vi "Finish.vi"   [LabVIEW 2015]
doc: "This VI is called just before exiting. It is expected to close I/O refnum, save collected data, etc."
uses:
  <vilib>/Rock Robotics/WPI/Utilities/WPI_GetSetVariantRefNum.vi
types:
  T1 = typedef "WPI_JoystickDevRef.ctl" = cluster{"Device":T2}
  T2 = typedef "WPI_JoystickDeviceEnum.ctl" = enum16{"USB 0", "USB 1", "USB 2", "USB 3", "USB 4", "USB 5"}
  T3 = typedef "WPI_CompressorDevRef.ctl" = cluster{"DevStatus":errorcluster, "Pneumatics Control Module":u8}
  T4 = typedef "WPI_EncoderDevRef.ctl" = cluster{"DevStatus":errorcluster, "EncoderIndex":T5, "CounterIndex":T6, "DistancePerCount":dbl, "Decoding Type":T7}
  T5 = typedef "FPGA_EncoderIdx.ctl" = enum8{"Enc 0", "Enc 1", "Enc 2", "Enc 3", "Enc 4", "Enc 5", "Enc 6", "Enc 7", "Invalid"}
  T6 = typedef "FPGA_CounterCtrSystemIndex.ctl" = enum8{"Ctr 0", "Ctr 1", "Ctr 2", "Ctr 3", "Ctr 4", "Ctr 5", "Ctr 6", "Ctr 7", "Invalid"}
  T7 = typedef "WPI_EncoderType.ctl" = enum16{"1x", "2x", "4x"}
  T8 = typedef "WPI_SolenoidDevRef.ctl" = cluster{"DevStatus":errorcluster, "Pneumatics Control Module":u8, "Forward Solenoid Channel":T9, "Reverse Solenoid Channel":T9}
  T9 = typedef "WPI_SolenoidChannel.ctl" = enum8{"Solenoid 0", "Solenoid 1", "Solenoid 2", "Solenoid 3", "Solenoid 4", "Solenoid 5", "Solenoid 6", "Solenoid 7", "Invalid"}
  T10 = typedef "WPI_ServoDeviceRef.ctl" = cluster{"DeviceStatus":errorcluster, "PWM Channel":T11, "DeadBand":T12}
  T11 = typedef "FPGA_DIOPWMChannel.ctl" = enum8{"PWM 0", "PWM 1", "PWM 2", "PWM 3", "PWM 4", "PWM 5", "PWM 6", "PWM 7", "PWM 8", "PWM 9", "PWM MXP 0", "PWM MXP 1", "PWM MXP 2", "PWM MXP 3", "PWM MXP 4", "PWM MXP 5", "PWM MXP 6", "PWM MXP 7", "PWM MXP 8", "PWM MXP 9", "Invalid"}
  T12 = typedef "WPI_PWMDeadband.ctl" = cluster{"Name":string, "maxPositivePwm":i32, "minPositivePwm":i32, "centerPwm":i32, "maxNegativePwm":i32, "minNegativePwm":i32, "angularRange":u16}
  T13 = typedef "WPI_RobotDriveDevRef.ctl" = cluster{"DevStatus":errorcluster, "Motors[]":T14[], "Square Inputs":bool, "Max Output":dbl}
  T14 = typedef "WPI_MotorControlDeviceRef.ctl" = cluster{"DeviceStatus":errorcluster, "Type":T15, "PWM":cluster{"PWM Channel":T11, "DeadBand":T12}, "CAN":cluster{"Device Number":u8, "Control Mode":T16, "Semaphore":T17, "Max Vout":dbl, "TalonSRX Control Mode":T18}, "Invert":bool}
  T15 = typedef "WPI_MotorControlType.ctl" = enum16{"PWM", "CAN", "CANTalonSRX"}
  T16 = typedef "WPI_CANJaguar_ControlMode.ctl" = enum8{"Percent VBus", "Current", "Speed", "Position", "Voltage"}
  T17 = typedef "Semaphore RefNum" = refnum<k1>
  T18 = typedef "WPI_CANTalonSRX_APIControlMode.ctl" = enum8{"Percent VBus", "Speed", "Position", "Slave", "Unchanged / Invalid", "Voltage Compensation", "Current", "Motion Profile"}
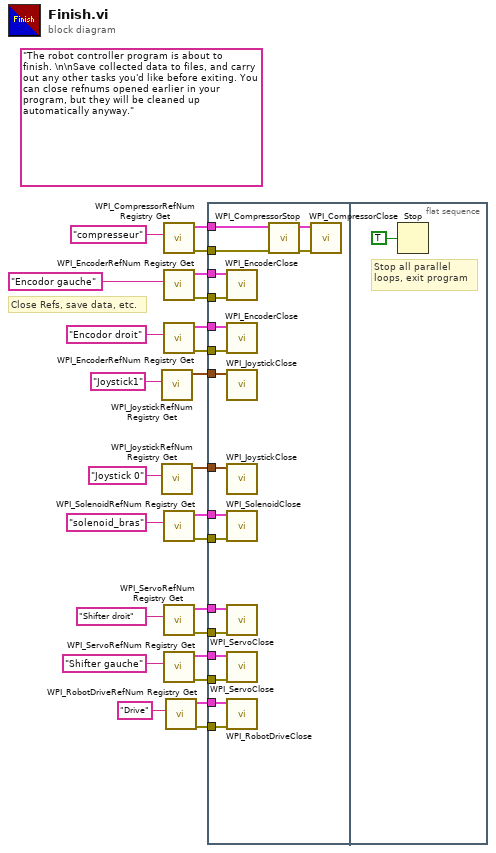
[diagram p0: block diagram]
diagram:
  (unwired) "The robot controller program is about to finish. \n\nSave collected data to files, and carry out any other tasks you'd like before exiting. You can close refnums opened earlier in your program, but they will be cleaned up automatically anyway."
  # "Close Refs, save data, etc."
  n1 = call <vilib>:"WPI_JoystickRefNum Registry Get.vi"("refnum name"="Joystick1") -> ("JoystickDevRef"=w16:T1)  [unwired: 1 in, 9 out]
  n2 = call <vilib>:"WPI_JoystickRefNum Registry Get.vi"("refnum name"="Joystick 0") -> ("JoystickDevRef"=w22:T1)  [unwired: 1 in, 9 out]
  n3 = call <vilib>:"WPI_CompressorRefNum Registry Get.vi"("refnum name"="compresseur") -> ("error out"=w12:errorcluster, "CompressorDevRef"=w13:T3)  [unwired: 9 in]
  n4 = call <vilib>:"WPI_EncoderRefNum Registry Get.vi"("refnum name"="Encodor gauche") -> ("error out"=w7:errorcluster, "EncoderDevRef"=w8:T4)  [unwired: 9 in]
  n5 = call <vilib>:"WPI_EncoderRefNum Registry Get.vi"("refnum name"="Encodor droit") -> ("error out"=w6:errorcluster, "EncoderDevRef"=w5:T4)  [unwired: 9 in]
  n6 = call <vilib>:"WPI_SolenoidRefNum Registry Get.vi"("refnum name"="solenoid_bras") -> ("error out"=w4:errorcluster, "SolenoidDevRef"=w15:T8)  [unwired: 9 in]
  n7 = call <vilib>:"WPI_ServoRefNum Registry Get.vi"("refnum name"="Shifter droit") -> ("error out"=w3:errorcluster, "ServoDeviceRef"=w21:T10)  [unwired: 9 in]
  n8 = call <vilib>:"WPI_ServoRefNum Registry Get.vi"("refnum name"="Shifter gauche") -> ("error out"=w2:errorcluster, "ServoDeviceRef"=w20:T10)  [unwired: 9 in]
  n9 = call <vilib>:"WPI_RobotDriveRefNum Registry Get.vi"("refnum name"="Drive") -> ("error out"=w1:errorcluster, "RobotDriveDevRef"=w23:T13)  [unwired: 1 in, 8 out]
  n10 = flat-sequence {
    tunnel: w23 -> [w43]
    tunnel: w22 -> [w42]
    tunnel: w21 -> [w41]
    tunnel: w20 -> [w40]
    tunnel: w16 -> [w39]
    tunnel: w15 -> [w38]
    tunnel: w13 -> [w35]
    tunnel: w12 -> [w34]
    tunnel: w8 -> [w33]
    tunnel: w7 -> [w32]
    tunnel: w6 -> [w31]
    tunnel: w5 -> [w30]
    tunnel: w4 -> [w29]
    tunnel: w3 -> [w28]
    tunnel: w2 -> [w27]
    tunnel: w1 -> [w26]
    frame #0 {
      n11 = call <vilib>:"WPI_EncoderClose.vi"("error in (no error)"=w32, "EncoderDevRef"=w33) -> ()  [unwired: 9 in, 1 out]
      n12 = call <vilib>:"WPI_EncoderClose.vi"("error in (no error)"=w31, "EncoderDevRef"=w30) -> ()  [unwired: 9 in, 1 out]
      n13 = call <vilib>:"WPI_JoystickClose.vi"("JoystickDevRef"=w39) -> ()  [unwired: 11 out]
      n14 = call <vilib>:"WPI_JoystickClose.vi"("JoystickDevRef"=w42) -> ()  [unwired: 11 out]
      n15 = call <vilib>:"WPI_SolenoidClose.vi"("error in (no error)"=w29, "SolenoidDevRef"=w38) -> ()  [unwired: 9 in, 1 out]
      n16 = call <vilib>:"WPI_ServoClose.vi"("error in (no error)"=w28, "ServoDeviceRef"=w41) -> ()  [unwired: 9 in, 1 out]
      n17 = call <vilib>:"WPI_ServoClose.vi"("error in (no error)"=w27, "ServoDeviceRef"=w40) -> ()  [unwired: 9 in, 1 out]
      n18 = call <vilib>:"WPI_RobotDriveClose.vi"("error in (no error)"=w26, "RobotDriveDevRef"=w43) -> ()  [unwired: 10 out]
      n19 = call <vilib>:"WPI_CompressorStop.vi"("error in (no error)"=w34, "CompressorDevRef"=w35) -> ("error out"=w37:errorcluster, "CompressorDevRef"=w36:T3)  [unwired: 8 in]
      n20 = call <vilib>:"WPI_CompressorClose.vi"("error in (no error)"=w37, "CompressorDevRef"=w36) -> ()  [unwired: 9 in, 1 out]
    }
    frame #1 {
      # "Stop all parallel\nloops, exit program"
      n21 = Stop(stop? (T)=TRUE ("Quit")) -> ()
    }
  }
